vi "LVClass_Image Get HASO sensor SN from image.vi"(0 "Image in":refnum<class "Image.lvclass">, 11 "error in (no error)":errorcluster) -> (4 "Image out":refnum<class "Image.lvclass">, 6 "haso_serial_number":string, 15 "error out":errorcluster)   [LabVIEW 2020, in "Image.lvclass"]
doc: "Get metadata from Image object.\n\n--------------------------------------------------------------------------------\n\n<B>ImageIn </B> : Image object.\n<B>ImageOut </B> : Image object.\n<B>haso_serial_number </B> : Haso serial number.\n<B>camera_serial_number </B> : Camera serial number.\n<B>exposure_time_applied </B> : Exposure duration applied (us).\n<B>exposure_time_requested </B> : Exposure duration requested (us).\n<B>gain </B> : Applied gain (SI).\n<B>nb_summed_images </B> : Number of summed images.\n<B>is_smearing_removed </B> : Smearing_removed.\n<B>is_background_removed </B> : Background_removed.\n<B>trigger_type </B> : Trigger mode.\n<B>time_stamp </B> : Date of the acquired Image.\n<B>max_level </B> : Max level value.\n<B>comments </B> : Comments.\n<B>ErrorIn </B> : Error\n<B>ErrorOut </B> : Error\n\n--------------------------------------------------------------------------------"
uses:
  Image.lvclass
  Image.lvclass/Image.ctl
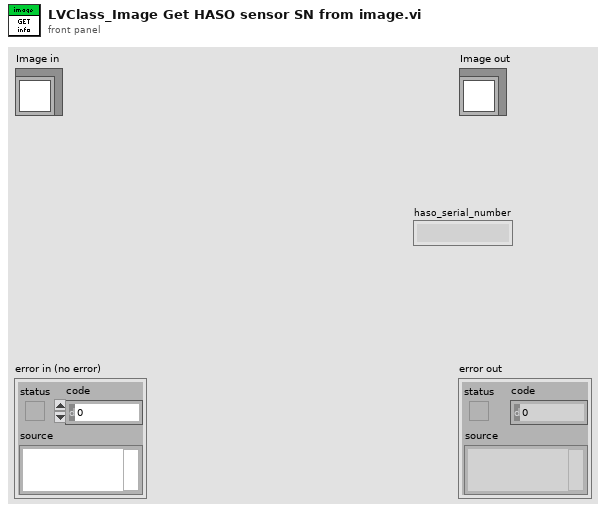
[diagram p1: front panel]
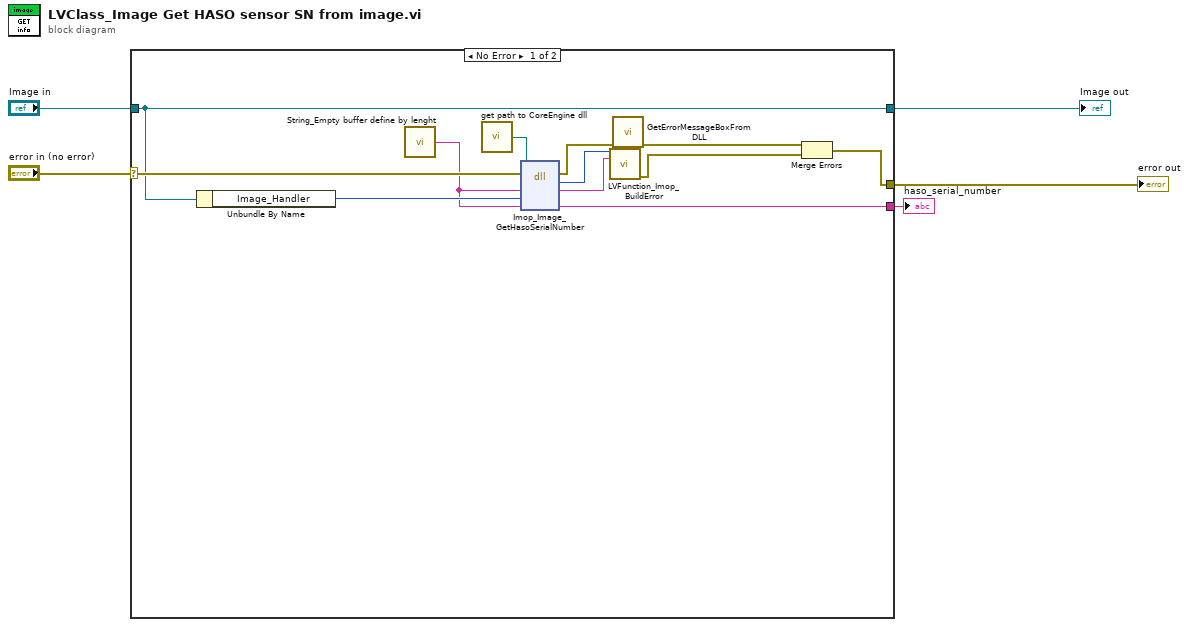
[diagram p0: block diagram]
diagram:
  n1 = case shown="No Error" "error in (no error)" {
    selector: "error in (no error)" -> [w9 w19]
    tunnel: [w10 w19] -> w4
    tunnel: [w8 w18] -> w2
    tunnel: "Image in" -> [w8 w18]
    tunnel: [w6 _] -> w1
    frame No Error {
      n2 = Unbundle By Name(w8) -> ("Image_Handler"=w17:i32)
      n3 = call "String_Empty buffer define by lenght.vi"() -> ("Empty buffer"=w7:string)  [unwired: 1 in]
      n4 = call "get path to CoreEngine dll.vi"() -> ("path to c_interface_vc100.dll"=w14:path)  [unwired: 12 in, 3 out]
      n5 = dll-call lib="D:/2_trunk/Soft_haso/ImOpCoreEngine4_LV2011/DLLs/ImopEngine4_vc100.dll" fn="Imop_Image_GetHasoSerialNumber"(path in=w14, error in=w9, "message"=w7, "Image compat"=w17, "haso_serial_number"=w7) -> (error out=w13:errorcluster, "return type"=w16:i32, "message"=w15:string, "haso_serial_number"=w6:string)  [unwired: 2 in, 1 out]
      n6 = call "LVFunction_Imop_BuildError.vi"("code"=w16, "String to Prepend to source (\"\")"=w15) -> ("error out"=w11:errorcluster)  [unwired: 13 in]
      n7 = call "GetErrorMessageBoxFromDLL.vi"("error IN"=w13) -> ("error OUT"=w12:errorcluster)  [unwired: 10 in]
      n8 = Merge Errors(w12, w11) -> (w10:errorcluster)
    }
    frame Error {
    }
  }
  "error out" <- w4
  "Image out" <- w2
  "haso_serial_number" <- w1
